vi "GEECS tcp parse single variable.vi"(11 "data in":string) -> (3 "variable value":string)   [LabVIEW 2020]
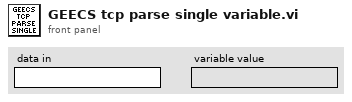
[diagram p1: front panel]
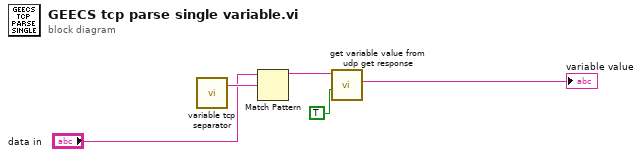
[diagram p0: block diagram]
diagram:
  n1 = call "variable tcp separator.vi"() -> ("variable separator"=w5:string)  [unwired: 3 in]
  n2 = Match Pattern(string="data in", regular expression=w5) -> (before substring=w2:string)  [unwired: 1 in, 3 out]
  n3 = call "get variable value from udp get response.vi"("tcp response"=TRUE, "slow get response or tcp response"=w2) -> ("variable value"=→"variable value":string)  [unwired: 3 in, 2 out]
